vi "Button Editor Config--constant.vi"() -> (3 "Button Editor Config":path)   [LabVIEW 2021, in "TSC Button Editor.lvclass"]
doc: "Constant VI to define the location of the button editor configuration file.\n\n<b>Code Developed By:</b>\nTechnology Service Corporation\n1983 S Liberty Drive\nBloomington, IN 47403\nwww.tsc.com/atcs\n\nDeveloper:\nDaniel Coons"
uses:
  TSC Button Editor.lvclass
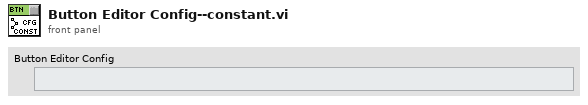
[diagram p1: front panel]
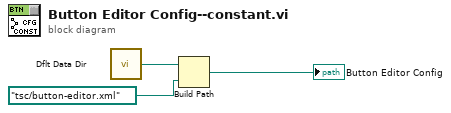
[diagram p0: block diagram]
diagram:
  n1 = call <vilib>:"Dflt Data Dir.vi"() -> ("App:Default Data Directory"=w1:path)
  n2 = Build Path(base path=w1, name or relative path=path "tsc/button-editor.xml") -> (appended path=→"Button Editor Config":path)
